vi "Create Analog Channel.vi"(6 "type":T1=enum."Output", 7 "default value":dbl, 8 "error in":errorcluster, 9 "index":i32, 10 "name":string, 11 "analog channel in":refnum<class "Analog Channel.lvclass">) -> (0 "error out":errorcluster, 3 "analog channel out":refnum<class "Analog Channel.lvclass">)   [LabVIEW 2020, in "Scan Engine Scripting.lvlib" / "Analog Channel.lvclass"]
uses:
  Analog Channel.lvclass
  Channel/Type.ctl
  Channel/Channel.lvclass
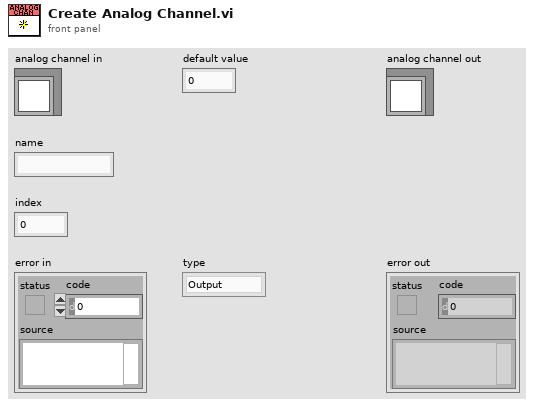
[diagram p1: front panel]
types:
  T1 = typedef "Scan Engine Scripting.lvlib/Channel.lvclass/Type.ctl" = enum16{"Input", "Output"}
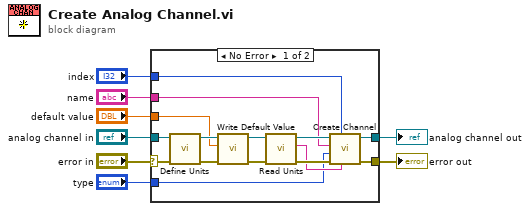
[diagram p0: block diagram]
diagram:
  n1 = case shown="No Error" "error in" {
    selector: "error in" -> [w16 w25]
    tunnel: [w15 w25] -> w7
    tunnel: [w13 w24] -> w5
    tunnel: "analog channel in" -> [w14 w24]
    tunnel: "default value" -> [w12 _]
    tunnel: "index" -> [w11 _]
    tunnel: "name" -> [w10 _]
    tunnel: "type" -> [w9 _]
    frame No Error {
      n2 = call-dynamic "Define Units.vi"("error in"=w16, "analog channel in"=w14) -> ("error out"=w22:errorcluster, "analog channel out"=w23:refnum<class "Analog Channel.lvclass">)  [unwired: 8 in]
      n3 = call-dynamic "Write Default Value.vi"("error in"=w22, "default value"=w12, "analog channel in"=w23) -> ("error out"=w20:errorcluster, "analog channel out"=w21:refnum<class "Analog Channel.lvclass">)  [unwired: 7 in]
      n4 = call-dynamic "Read Units.vi"("error in"=w20, "channel in"=w21) -> ("error out"=w18:errorcluster, "units"=w17:string, "channel out"=w19:refnum<class "Analog Channel.lvclass">)  [unwired: 7 in]
      n5 = call-dynamic "Create Channel.vi"("units"=w17, "index"=w11, "error in"=w18, "type"=w9, "name"=w10, "channel in"=w19) -> ("error out"=w15:errorcluster, "channel out"=w13:refnum<class "Analog Channel.lvclass">)  [unwired: 4 in]
    }
    frame Error {
    }
  }
  "error out" <- w7
  "analog channel out" <- w5
